vi "Create Slewing Test Waveform.vi"(11 "Model in":refnum<class "Model.lvclass">) -> (2 "Waveform":refnum<class "Waveform.lvclass">, 3 "Model out":refnum<class "Model.lvclass">)   [LabVIEW 2016]
uses:
  Typedefs/WaveformTypes.ctl
  Typedefs/WaveformSettings.ctl
  Model/Waveforms/Waveform Factory/Waveform Factory.lvclass
  Model/Model/Model.lvclass
  Model/Waveforms/Waveform/Waveform.lvclass
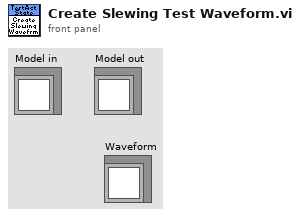
[diagram p1: front panel]
types:
  T1 = typedef "WaveformTypes.ctl" = enum16{"Sine", "Triangle", "Square", "Sawtooth", "Chirp", "Gaussian", "Trapezoid", "Constant"}
  T2 = typedef "WaveformSettings.ctl" = cluster{"Sample Count":u32, "Amplitude":dbl, "Offset":dbl, "Frequency":dbl[unit], "Waveform":T1, "F1":dbl[unit], "F2":dbl[unit], "Duty Cycle":dbl, "ILC Rate":dbl[unit], "Ramp Time":dbl[unit], "Hold Time":dbl[unit], "Settling Time":dbl[unit], "Delay":dbl[unit]}
  T3 = typedef "SlewingTestSettings.ctl" = cluster{"Max Force Error (N)":dbl, "Max Moment (NM)":dbl, "Amplitude (N)":dbl, "Max Instance Force Error (N)":dbl, "Ramp Time (s)":dbl, "Hold Time (s)":dbl, "Settling Time (s)":dbl}
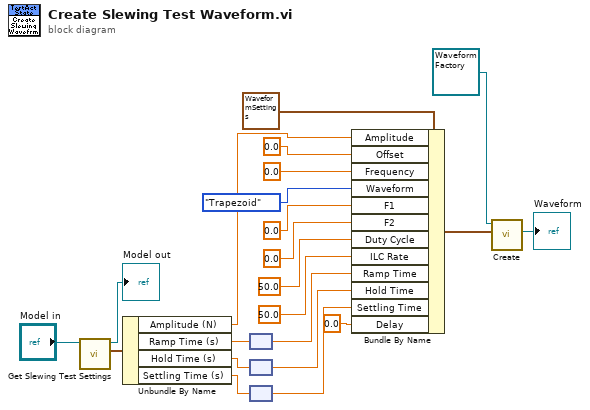
[diagram p0: block diagram]
diagram:
  n1 = call "Get Slewing Test Settings.vi"("Model in"="Model in") -> ("Slewing Test Settings"=w14:T3, "Model out"=→"Model out":refnum<class "Model.lvclass">)  [unwired: 9 in]
  n2 = Unbundle By Name(w14) -> ("Amplitude (N)"=w15:dbl, "Ramp Time (s)"=w7:dbl, "Hold Time (s)"=w6:dbl, "Settling Time (s)"=w5:dbl)
  n3 = node(w7) -> (w2:dbl[unit])
  n4 = node(w6) -> (w3:dbl[unit])
  n5 = node(w5) -> (w4:dbl[unit])
  n6 = Bundle By Name(cluster=T2 {"Sample Count"=0, "Amplitude"=0.0, "Offset"=0.0, "Frequency"=0.0, "Waveform"=enum."Sine", "F1"=0.0, "F2"=0.0, "Duty Cycle"=0.0, "ILC Rate"=0.0, "Ramp Time"=0.0, "Hold Time"=0.0, "Settling Time"=0.0, "Delay"=0.0} ("Waveform Settings"), "Amplitude"=w15, "Offset"=0.0, "Frequency"=dbl[unit] 0.0, "Waveform"=WaveformTypes."Trapezoid", "F1"=dbl[unit] 0.0, "F2"=dbl[unit] 0.0, "Duty Cycle"=50.0, "ILC Rate"=dbl[unit] 50.0, "Ramp Time"=w2, "Hold Time"=w3, "Settling Time"=w4, "Delay"=dbl[unit] 0.0) -> (w9:T2)
  n7 = call-dynamic "Create.vi"("Waveform Settings"=w9, "Waveform Factory in"=refnum<class "Waveform Factory.lvclass"> refnum ("Waveform Factory.lvclass")) -> ("Waveform"=→"Waveform":refnum<class "Waveform.lvclass">)  [unwired: 7 in, 2 out]
